vi "JsonParseConnectionInfo.vi"(8 "error in (no error)":errorcluster, 11 "JSON string":string) -> (0 "error out":errorcluster, 3 "connection info":T1)   [LabVIEW 2017, in "ServerComm.lvlib"]
uses:
  <vilib>/addons/InsightCM/Devices/Shared/Common/ServerComm/ServerComm.lvlib
  <vilib>/addons/InsightCM/MessageBus/Base/controls/ConnectionInfo.ctl
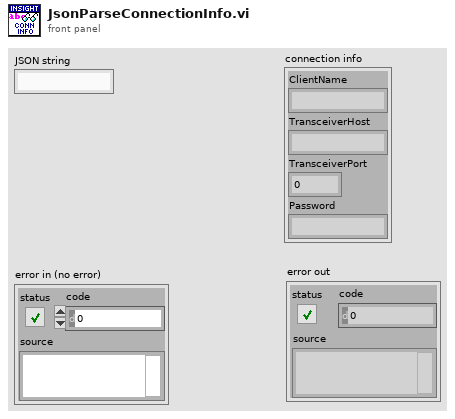
[diagram p1: front panel]
types:
  T1 = typedef "ConnectionInfo.ctl" = cluster{"ClientName":string, "TransceiverHost":string, "TransceiverPort":u16, "Password":string}
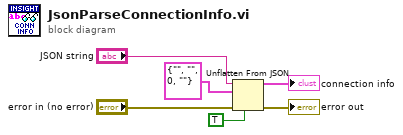
[diagram p0: block diagram]
diagram:
  n1 = Unflatten From JSON(JSON string="JSON string", type and defaults=T1 {"ClientName"="", "TransceiverHost"="", "TransceiverPort"=0, "Password"=""} ("ConnInfo"), default null elements? (F)=TRUE, error in (no error)="error in (no error)") -> (value=→"connection info":T1, error out=→"error out":errorcluster)  [unwired: 3 in]
